vi "getState.vi"(8 "error in (no error)":errorcluster, 11 "SudukuState in":refnum<class "SudokuState.lvclass">) -> (0 "error out":errorcluster, 2 "State":cluster{"Value":i32, "Options":i32[]}[][](array[cluster]), 3 "SudukuState out":refnum<class "SudokuState.lvclass">)   [LabVIEW 2010, in "SudokuState.lvclass"]
uses:
  SudokuState.lvclass
  SudokuState.lvclass/SudokuState.ctl
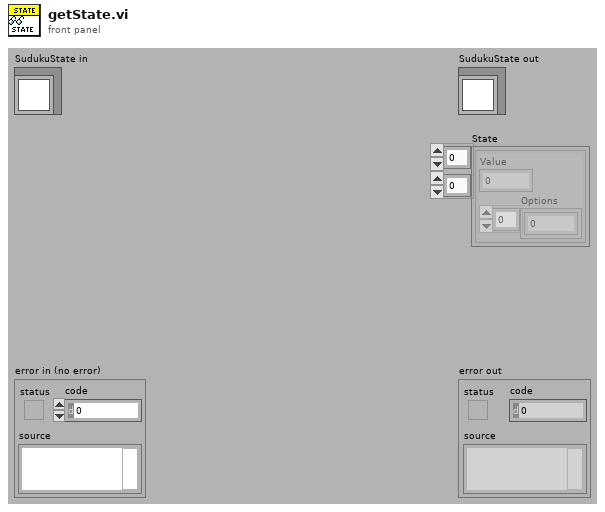
[diagram p1: front panel]
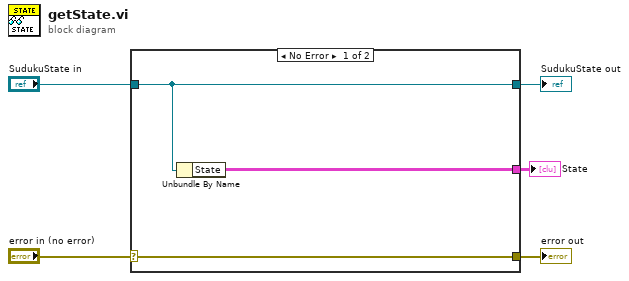
[diagram p0: block diagram]
diagram:
  n1 = case shown="No Error" "error in (no error)" {
    selector: "error in (no error)" -> [w8 w9]
    tunnel: [w8 w9] -> w4
    tunnel: [w7 w10] -> w2
    tunnel: "SudukuState in" -> [w7 w10]
    tunnel: [w6 _] -> w1
    frame No Error {
      n2 = Unbundle By Name(w7) -> ("State"=w6:cluster{"Value":i32, "Options":i32[]}[][])
    }
    frame Error {
    }
  }
  "error out" <- w4
  "SudukuState out" <- w2
  "State" <- w1
